vi "Name Label Color Read.vi"(8 "error in (no error)":errorcluster, 11 "3D Plot.lvclass in":refnum<class "3D Plot.lvclass">) -> (0 "error out":errorcluster, 1 "Caption Color":u32, 3 "3D Plot.lvclass out":refnum<class "3D Plot.lvclass">)   [LabVIEW 2020, in "3D Plot.lvclass"]
uses:
  <vilib>/Math Plots/3D Math Plots/3D Plot/3D Plot/3D Plot.lvclass
  <vilib>/Math Plots/3D Math Plots/3D Plot/3D Plot/3D Plot.lvclass/3D Plot.ctl
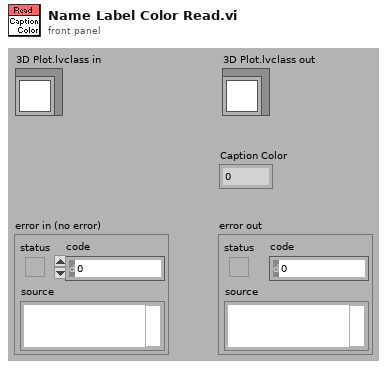
[diagram p1: front panel]
types:
  T1 = cluster{"Caption Color X":u32, "Caption Color Y":u32, "Caption Color Z":u32}
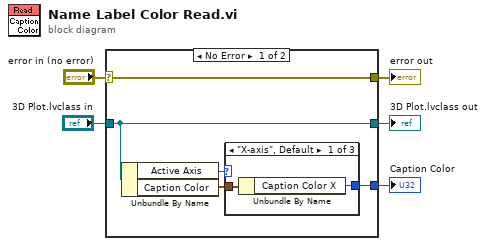
[diagram p0: block diagram]
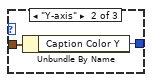
[diagram p2: hidden frame]
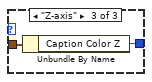
[diagram p3: hidden frame]
diagram:
  n1 = case shown="No Error" "error in (no error)" {
    selector: "error in (no error)" -> [w7 w17]
    tunnel: [w10 _] -> w5
    tunnel: "3D Plot.lvclass in" -> [w6 w18]
    tunnel: [w7 w17] -> w2
    tunnel: [w6 w18] -> w1
    frame No Error {
      n2 = Unbundle By Name(w6) -> ("Active Axis"=w8:enum16{"X-axis", "Y-axis", "Z-axis"}, "Caption Color"=w9:T1)
      n3 = case shown="\"X-axis\", Default" w8 {
        tunnel: w9 -> [w11 w14 w16]
        tunnel: [w12 w13 w15] -> w10
        frame "X-axis", Default {
          n4 = Unbundle By Name(w11) -> ("Caption Color X"=w12:u32)
        }
        frame "Y-axis" {
          n5 = Unbundle By Name(w14) -> ("Caption Color Y"=w13:u32)
        }
        frame "Z-axis" {
          n6 = Unbundle By Name(w16) -> ("Caption Color Z"=w15:u32)
        }
      }
    }
    frame Error {
    }
  }
  "error out" <- w2
  "Caption Color" <- w5
  "3D Plot.lvclass out" <- w1
